vi "Write  InI.vi"(8 "error in (no error)":errorcluster, 9 "value":string, 10 "key":string="key", 11 "section":string="Section") -> (0 "error out":errorcluster, 3 "file path":path)   [LabVIEW 2020]
uses:
  a0625001-b31d-4342-89f0-0b96323064cc.vi
  <vilib>/Utility/config.llb/Write Key (String).vi
  <vilib>/Utility/config.llb/NI_LVConfig.lvlib
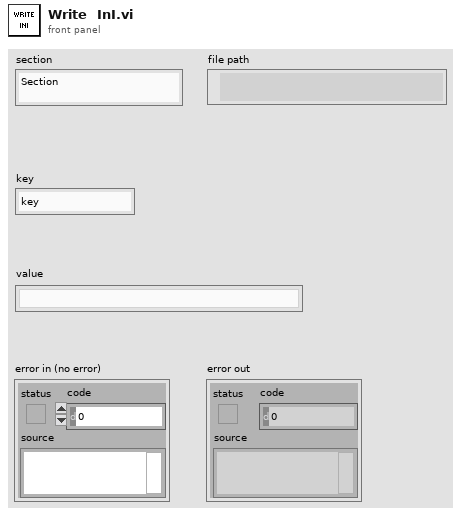
[diagram p1: front panel]
types:
  T1 = typedef "NI_LVConfig.lvlib/Config Data RefNum.ctl" = refnum<k1>
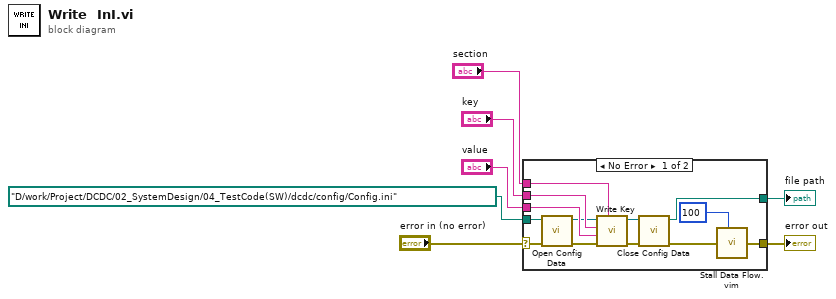
[diagram p0: block diagram]
diagram:
  n1 = case shown="No Error" "error in (no error)" {
    selector: "error in (no error)" -> [w19 w22]
    tunnel: "key" -> [w17 _]
    tunnel: "section" -> [w16 _]
    tunnel: path "D:/work/Project/DCDC/02_SystemDesign/04_TestCode(SW)/dcdc/config/Config.ini" ("appended path") -> [w20 w21]
    tunnel: [w11 w22] -> w4
    tunnel: "value" -> [w15 _]
    tunnel: [w8 w21] -> w2
    frame No Error {
      n2 = call <vilib>:"Open Config Data.vi"("error in (no error)"=w19, "configuration file path"=w20) -> ("error out"=w18:errorcluster, "refnum"=w14:T1)  [unwired: 7 in, 1 out]
      n3 = call-poly <vilib>:"Write Key.vi"("section"=w16, "error in (no error)"=w18, "value"=w15, "key"=w17, "refnum"=w14) -> ("error out"=w13:errorcluster, "refnum out"=w12:T1)  [unwired: 4 in, 1 out]
      n4 = call <vilib>:"Close Config Data.vi"("error in (no error)"=w13, "refnum"=w12) -> ("error out"=w10:errorcluster, "file path"=w8:path)  [unwired: 8 in]
      n5 = call "Stall Data Flow.vim"("value in"=w10, "milliseconds to wait"=u32 100) -> ("value out"=w11:errorcluster)  [unwired: 1 out]
    }
    frame Error {
    }
  }
  "error out" <- w4
  "file path" <- w2
